vi "Turtlesim Subscribe.vi"() -> ()   [LabVIEW 2015]
uses:
  ROS/Code/Console/Servers/ServerSubs/TopicDef.ctl
  ROS/Code/SubVIs/_ROSDirection.ctl
panel:
  out "Twist":T1
  out "error out":errorcluster
  in  "stop":bool
  # "This VI is meant to be used with the turtlesim example in ROS. Before running this VI, follow the instructions at http://wiki.ros.org/ROS/Tutorials/UnderstandingTopics"
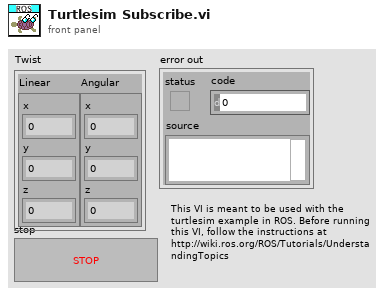
[diagram p1: front panel]
types:
  T1 = cluster{"Linear":cluster{"x":dbl, "y":dbl, "z":dbl}, "Angular":cluster{"x":dbl, "y":dbl, "z":dbl}}
  T2 = typedef "TopicDef.ctl" = cluster{"Topic":string, "Type":string, "Action":T3, "Update (ms)":u16, "queue size":u16}
  T3 = typedef "_ROSDirection.ctl" = enum16{"Node", "Publisher", "Subscriber", "ServiceClient", "ServiceProvider"}
  T4 = typedef "_ROSControl.ctl" = cluster{"topic port":u16, "Node":string, "topic":string, "type":string, "node port":u16, "error ":errorcluster, "Direction":T3, "Update (ms)":u16, "FIFO size":u16}
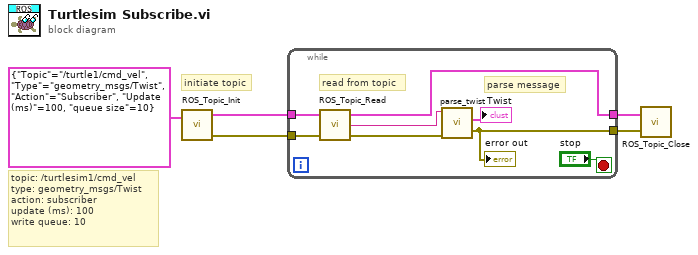
[diagram p0: block diagram]
diagram:
  # "initiate topic"
  # "topic: /turtlesim1/cmd_vel\ntype: geometry_msgs/Twist\naction: subscriber\nupdate (ms): 100\nwrite queue: 10"
  n1 = call "ROS_Topic_Init.vi"("Definitions"=T2 {"Topic"="/turtle1/cmd_vel", "Type"="geometry_msgs/Twist", "Action"=enum."Subscriber", "Update (ms)"=100, "queue size"=10}) -> ("ROS out"=w4:T4, "error out"=w3:errorcluster)  [unwired: 2 in]
  n2 = while {
    tunnel: w4 -> [w13]
    tunnel: w3 -> [w12]
    tunnel: [w10] -> w2
    tunnel: [w7] -> w1
    stop <- "stop" stop-if-true
    # "parse message"
    # "read from topic"
    n3 = call "ROS_Topic_Read.vi"("error in (no error)"=w12, "ROS in"=w13) -> ("error out"=w8:errorcluster, "Reply"=w9:string, "ROS out"=w10:T4)  [unwired: 1 in]
    n4 = call "parse_twist.vi"("error in"=w8, "msg in"=w9) -> ("error out"=w7:errorcluster, "Twist"=→"Twist":T1)  [unwired: 3 in, 1 out]
    "error out" <- w7
  }
  n5 = call "ROS_Topic_Close.vi"("error in"=w1, "ROS in"=w2) -> ()  [unwired: 2 in, 1 out]
